vi "S2DS_ErrorCheckingInY.vi"(0 "Scan parameters in":T1 {"Y data taking" items=["in both direction", "in up direction only", "in down direction only"]; "X data taking" items=["in both direction", "in up direction only", "in down direction only"]}) -> (1 "Error string out":string, 2 "Error? (out)":bool)   [LabVIEW 2025]
uses:
  TYPE DEFS/S2DS_Sweep Info.ctl
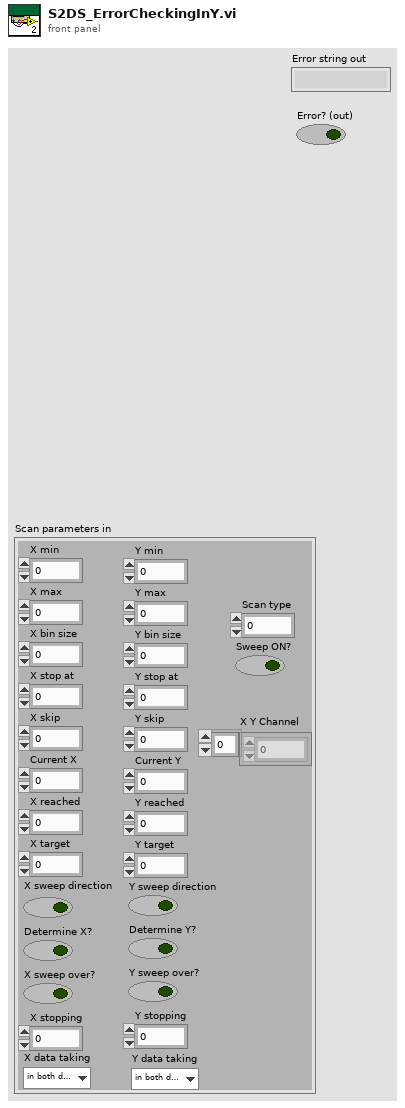
[diagram p1: front panel]
types:
  T1 = typedef "S2DS_Sweep Info.ctl" = cluster{"X min":ext, "X max":dbl, "Y min":dbl, "Y max":dbl, "X bin size":dbl, "Y bin size":dbl, "X stop at":dbl, "Y stop at":dbl, "X skip":u64, "Y skip":u64, "Current X":dbl, "Current Y":dbl, "X reached":i32, "Y reached":i32, "X target":dbl, "Y target":dbl, "Sweep ON?":bool, "X sweep direction":bool, "Y sweep direction":bool, "Determine X?":bool, "Determine Y?":bool, "X sweep over?":bool, "Y sweep over?":bool, "Scan type":i32, "X stopping":i32, "Y stopping":i32, "X Y Channel":u16[], "X data taking":u16, "Y data taking":u16}
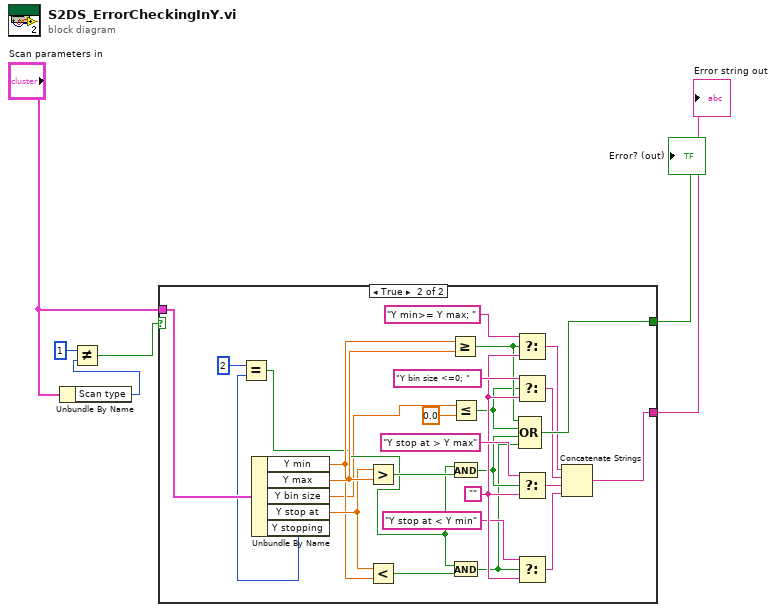
[diagram p0: block diagram]
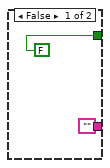
[diagram p2: hidden frame]
diagram:
  n1 = Unbundle By Name("Scan parameters in") -> ("Scan type"=w5:i32)
  n2 = Not Equal?(x=1, y=w5) -> (x != y?=w4:bool)
  n3 = case shown="True" w4 {
    tunnel: "Scan parameters in" -> [_ w34]
    tunnel: [FALSE w19] -> w1
    tunnel: ["" w14] -> w2
    frame False {
    }
    frame True {
      w25 = ""
      n4 = Unbundle By Name(w34) -> ("Y min"=w27:dbl, "Y max"=w31:dbl, "Y bin size"=w10:dbl, "Y stop at"=w28:dbl, "Y stopping"=w12:i32)
      n5 = Equal?(x=2, y=w12) -> (x = y?=w11:bool)
      n6 = Greater?(x=w28, y=w31) -> (0:w30:bool)
      n7 = Less?(x=w28, y=w27) -> (x < y?=w26:bool)
      n8 = Greater Or Equal?(x=w27, y=w31) -> (x >= y?=w23:bool)
      n9 = Less Or Equal?(x=w10, y=0.0) -> (x <= y?=w22:bool)
      n10 = And(x=w11, y=w30) -> (x .and. y?=w21:bool)
      n11 = And(x=w11, y=w26) -> (x .and. y?=w20:bool)
      n12 = Select(t="Y min>= Y max; ", s=w23, f=w25) -> (s? t:f=w18:string)
      n13 = Select(t="Y bin size <=0; ", s=w22, f=w25) -> (s? t:f=w17:string)
      n14 = Select(t="Y stop at > Y max", s=w21, f=w25) -> (s? t:f=w16:string)
      n15 = Select(t="Y stop at < Y min", s=w20, f=w25) -> (s? t:f=w15:string)
      n16 = Compound Arithmetic op=OR(w23, w22, w21, w20) -> (w19:bool)
      n17 = Concatenate Strings(w18, w17, w16, w15) -> (w14:string)
    }
  }
  "Error string out" <- w2
  "Error? (out)" <- w1
